vi "ToRing.vi"(8 "error in":errorcluster, 11 "Ring in":refnum<class "Generic.lvclass">) -> (0 "error out":errorcluster, 3 "Ring out":refnum<class "Ring.lvclass">)   [LabVIEW 2014, in "Raspberry Pi Compatible Compiler for LabVIEW.lvlib" / "Ring.lvclass"]
uses:
  Ring.lvclass
  Generic/Generic.lvclass
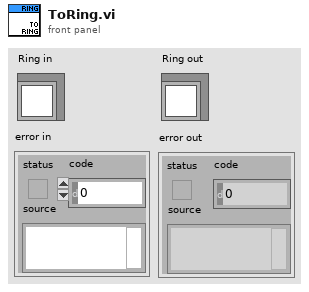
[diagram p1: front panel]
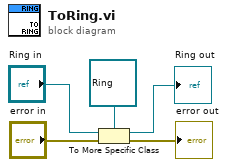
[diagram p0: block diagram]
diagram:
  n1 = To More Specific Class(target class=refnum<class "Ring.lvclass"> refnum ("Ring in"), reference="Ring in", error in="error in") -> (specific class reference=→"Ring out":refnum<class "Ring.lvclass">, error out=→"error out":errorcluster)
